vi "Client Cancel Call Context.vi"(8 "error in":errorcluster, 11 "Context ID in":T1) -> (0 "error out":errorcluster, 3 "Context ID out":T1)   [LabVIEW 2019, in "grpc-lvsupport.lvlib"]
uses:
  grpc-lvsupport.lvlib
  Shared/grpcId.ctl
  <vilib>/Utility/error.llb/Error Cluster From Error Code.vi
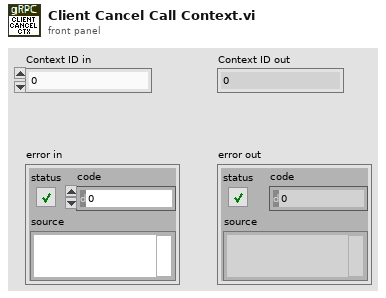
[diagram p1: front panel]
types:
  T1 = typedef "grpc-lvsupport.lvlib/grpcId.ctl" = u64
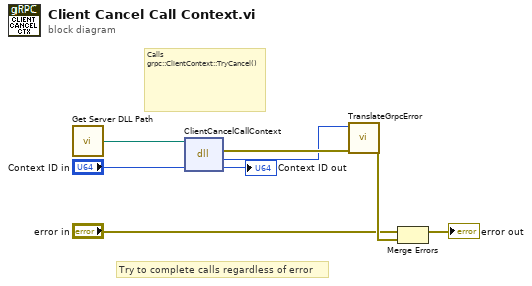
[diagram p0: block diagram]
diagram:
  # "Calls \ngrpc::ClientContext::TryCancel()"
  # "Try to complete calls regardless of error"
  n1 = call "Get Server DLL Path.vi"() -> ("server dll path"=w6:path)
  n2 = dll-call lib="?" fn="ClientCancelCallContext"(path in=w6, "contextId"="Context ID in") -> (error out=w8:errorcluster, "return type"=w5:i32, "contextId"=→"Context ID out":u64)  [unwired: 2 in, 1 out]
  n3 = call "TranslateGrpcError.vi"("error in"=w8, "Error Code"=w5) -> ("error out"=w4:errorcluster)  [unwired: 9 in]
  n4 = Merge Errors("error in", w4) -> (→"error out":errorcluster)
